vi "arduinoValveArrayToByte.vi"(1 "MSB first":bool, 2 "valve data open":bool[](array[boolean])=[TRUE, FALSE, FALSE, FALSE, FALSE, FALSE, FALSE, FALSE]) -> (0 "output":u8)   [LabVIEW 2012]
panel:
  out "Array":i32[](array[numeric])
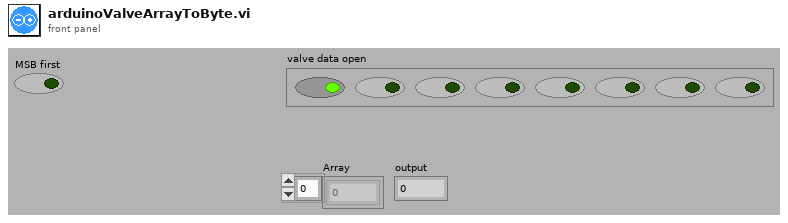
[diagram p1: front panel]
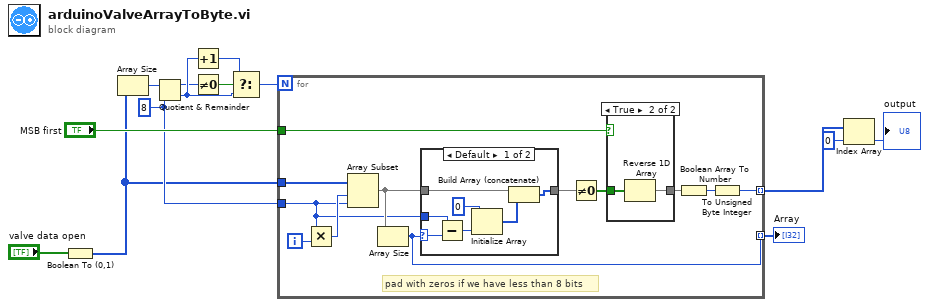
[diagram p0: block diagram]
diagram:
  w7 = 8 ("Numeric")
  n1 = Boolean To (0,1)(Boolean="valve data open") -> (0, 1=w1:i16[])
  n2 = Array Size(array=w1) -> (size(s)=w6:i32)
  n3 = Quotient & Remainder(x=w6, y=w7) -> (x-y*floor(x/y)=w10:i32, floor(x/y)=w13:i32)
  n4 = Increment(x=w13) -> (x+1=w14:i32)
  n5 = Not Equal To 0?(x=w10) -> (x != 0?=w11:bool)
  n6 = Select(t=w14, s=w11, f=w13) -> (s? t:f=w12:i32)
  n7 = for {
    N: w12 -> [_]
    tunnel: w1 -> [w26]
    tunnel: w7 -> [w15]
    tunnel: [w20] -> w5 mode=indexing
    tunnel: "MSB first" -> [w19]
    tunnel: [w18] -> w9 mode=indexing
    i -> [w25]
    # "pad with zeros if we have less than 8 bits"
    n8 = Multiply(x=w15, y=w25) -> (x*y=w24:i32)
    n9 = Array Subset(array=w26, index=w24, length=w15) -> (w17:i16[])
    n10 = Array Size(array=w17) -> (size(s)=w18:i32)
    n11 = case shown="Default" w18 {
      selector: w18 -> [w31 _]
      tunnel: w17 -> [w33 w34]
      tunnel: [w32 w34] -> w16
      tunnel: w15 -> [w30 _]
      frame Default {
        n12 = Subtract(x=w30, y=w31) -> (x-y=w29:i32)
        n13 = Initialize Array(0 ("Numeric"), w29) -> (w27:i32[])
        n14 = Build Array (concatenate)(w33, w27) -> (w32:i32[])
      }
      frame 16 {
      }
    }
    n15 = Not Equal To 0?(x=w16) -> (x != 0?=w22:bool[])
    n16 = case shown="True" w19 {
      tunnel: w22 -> [w35 w37]
      tunnel: [w35 w36] -> w21
      frame False {
      }
      frame True {
        n17 = Reverse 1D Array(array=w37) -> (reversed array=w36:bool[])
      }
    }
    n18 = Boolean Array To Number(Boolean array=w21) -> (number=w23:u32)
    n19 = To Unsigned Byte Integer(number=w23) -> (unsigned 8bit integer=w20:u8)
  }
  "Array" <- w9
  n20 = Index Array(array=w5, index=0) -> (element=→"output":u8)
